vi "S2C_VLFT10_Proc_Audio.vi"(8 "Error In":errorcluster) -> (0 "Error Out":errorcluster, 3 "Result":string)   [LabVIEW 2015]
uses:
  Fornax/VIs/PolyDriver/Typedefs/AudioSequence.ctl
  Fornax/VIs/PolyDriver/Typedefs/AudioMode.ctl
  Fornax/VIs/PolyDriver/Typedefs/AudioPriority.ctl
panel:
  in  "No":bool
  in  "Yes":bool
  # "Can you hear Audio Playing?"
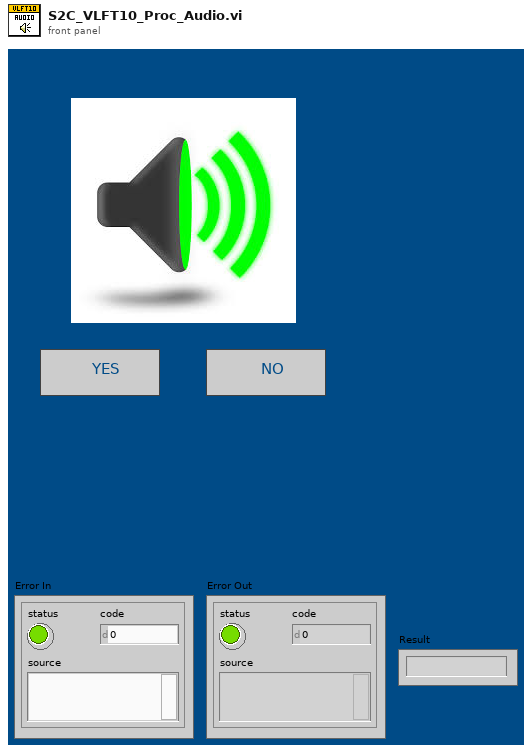
[diagram p1: front panel]
types:
  T1 = cluster{"Driver":string, "Command":string, "Return":string, "Parameters":string, "Timeout":dbl}
  T2 = typedef "AudioSequence.ctl" = i16
  T3 = typedef "AudioMode.ctl" = i16
  T4 = typedef "AudioPriority.ctl" = i16
  T5 = cluster{"Partition":string, "Message":string, "M_AudioSequence":T2, "M_PlayMode":T3, "M_Priority":T4, "M_OverrideSeqVolume":bool, "M_Volume":i32}
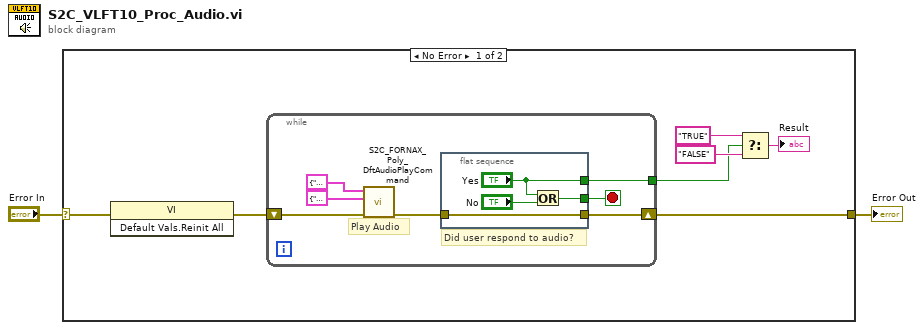
[diagram p0: block diagram]
diagram:
  n1 = case shown="No Error" "Error In" {
    selector: "Error In" -> [w4 w21]
    tunnel: [w6 w21] -> w2
    frame No Error {
      n2 = invoke class="VI" method="Default Vals.Reinit All"(error in=w4) -> (error out=w3:errorcluster)  [unwired: 2 in, 2 out]
      n3 = while {
        shift-right: [w11] -> w6
        shift-left: w3 -> [w16]
        tunnel: [w10] -> w5
        stop <- w14 stop-if-true
        # "Did user respond to audio?"
        # "Play Audio"
        n4 = call "S2C_FORNAX_Poly_DftAudioPlayCommand.vi"("Error In"=w16, "DftAudioPlayCommand"=T5 {"Partition"="Default", "Message"="DftAudioPlayCommand", "M_AudioSequence"=1, "M_PlayMode"=3, "M_Priority"=0, "M_OverrideSeqVolume"=FALSE, "M_Volume"=0}, "Settings"=T1 {"Driver"="Fornax", "Command"="DftAudioPlayCommand", "Return"="ErrorStatus", "Parameters"="", "Timeout"=1.0}) -> ("Error Out"=w12:errorcluster)  [unwired: 7 in, 1 out]
        n5 = flat-sequence {
          tunnel: [w19] -> w14
          tunnel: w12 -> [w18]
          tunnel: [w18] -> w11
          tunnel: ["Yes"] -> w10
          frame #0 {
            n6 = Or(x="Yes", y="No") -> (x .or. y?=w19:bool)
          }
        }
      }
      n7 = Select(t="TRUE", s=w5, f="FALSE") -> (s? t:f=→"Result":string)
    }
    frame Error {
    }
  }
  "Error Out" <- w2
